vi "Initialize.vi"(8 "error in (no error)":errorcluster, 9 "Reset (True)":bool=TRUE, 10 "ID Query (True)":bool=TRUE, 11 "VISA resource name":refnum<visa-resource-name>) -> (0 "error out":errorcluster, 3 "VISA resource name out":refnum<visa-resource-name>)   [LabVIEW 2015, in "ZhiYuan ZDS Series for TCP.lvlib"]
doc: "Establishes communication with the instrument and optionally performs an instrument identification query and/or an instrument reset. It also places the instrument in a default state needed for other instrument driver operations. Therefore, call this VI before calling other instrument driver VIs for this instrument. Generally, you need to call the Initialize VI only once at the beginning of an application."
uses:
  ZhiYuan ZDS Series for TCP.lvlib
panel:
  # "(c) 2012 National Instruments.  ALL RIGHTS RESERVED."
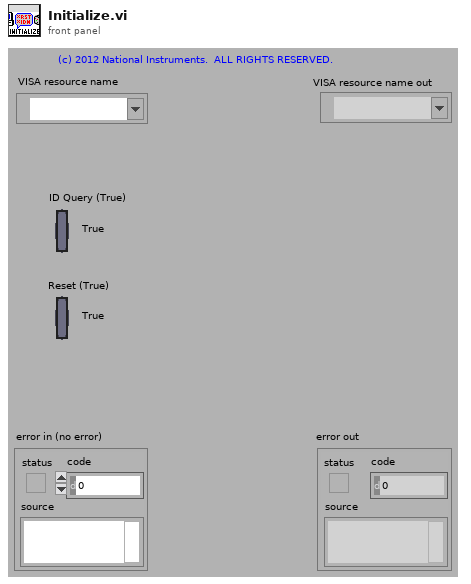
[diagram p1: front panel]
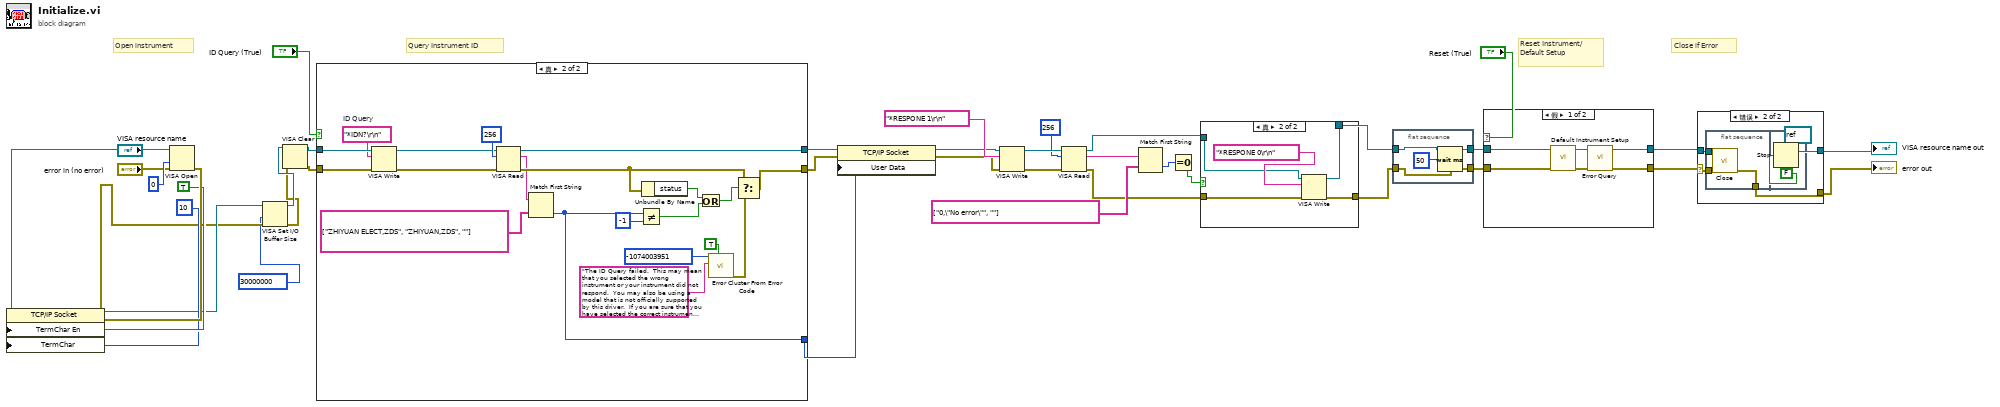
[diagram p0: block diagram]
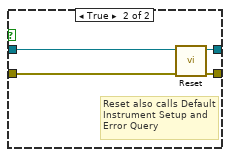
[diagram p4: hidden frame]
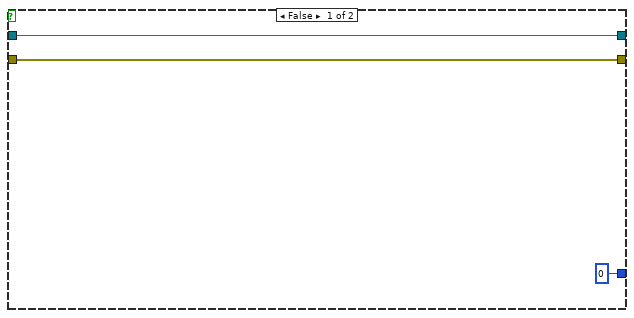
[diagram p5: hidden frame]
diagram:
  # "Close if Error"
  # "Query Instrument ID"
  # "Reset Instrument/\nDefault Setup"
  # "Open instrument"
  n1 = VISA Open(access mode=u32 0, error in (no error)="error in (no error)", VISA resource name="VISA resource name") -> (VISA resource name=w31:refnum<visa-resource-name>, error out=w30:errorcluster)  [unwired: 2 in]
  n2 = property class="TCP/IP Socket"(reference=w31, error in=w30, "TermChar En"=TRUE ("Message Based Settings:Termination Character Enable"), "TermChar"=u8 10 ("Message Based Settings:Termination Character")) -> (reference out=w23:refnum<visa-resource-name>, error out=w21:errorcluster)
  n3 = VISA Set I/O Buffer Size(VISA resource name=w23, size (4096)=30000000, error in (no error)=w21) -> (VISA resource name out=w22:refnum<visa-resource-name>, error out=w20:errorcluster)  [unwired: 1 in]
  n4 = VISA Clear(VISA resource name=w22, error in (no error)=w20) -> (VISA resource name out=w36:refnum<visa-resource-name>, error out=w35:errorcluster)
  n5 = case shown="真" "ID Query (True)" {
    tunnel: [w41 w62] -> w33
    tunnel: [w42 w59] -> w34
    tunnel: w36 -> [w42 w60]
    tunnel: w35 -> [w41 w61]
    tunnel: [0 ("index") w45] -> w32
    frame False {
    }
    frame True {
      w57 = "*IDN?\r\n"  # ID Query
      n6 = VISA Write(VISA resource name=w60, write buffer=w57, error in (no error)=w61) -> (VISA resource name out=w44:refnum<visa-resource-name>, error out=w43:errorcluster)  [unwired: 1 out]
      n7 = VISA Read(VISA resource name=w44, byte count=u32 256, error in (no error)=w43) -> (VISA resource name out=w59:refnum<visa-resource-name>, read buffer=w47:string, error out=w52:errorcluster)  [unwired: 1 out]
      n8 = Match First String(2:string[] ["ZHIYUAN ELECT,ZDS", "ZHIYUAN,ZDS", ""], 3:w47) -> (0:w45:i32)  [unwired: 1 out]
      n9 = Not Equal?(x=w45, y=-1) -> (x != y?=w50:bool)
      n10 = Unbundle By Name(w52) -> ("status"=w51:bool)
      n11 = Or(x=w51, y=w50) -> (x .or. y?=w49:bool)
      n12 = call <vilib>:"Error Cluster From Error Code.vi"("show call chain? (False)"=TRUE, "error message (\"\")"="The ID Query failed.  This may mean that you selected the wrong instrument or your instrument did not respond.  You may also be using a model that is not officially supported by this driver.  If you are sure that you have selected the correct instrument and it is responding, try disabling the ID Query." ("Source (VI Name)"), "error code (0)"=-1074003951 ("Code")) -> ("error out"=w56:errorcluster)  [unwired: 6 in]
      n13 = Select(t=w52, s=w49, f=w56) -> (s? t:f=w62:errorcluster)
    }
  }
  n14 = property on="Property Node" class="TCP/IP Socket"(reference=w34, error in=w33, "User Data"=w32) -> (reference out=w8:refnum<visa-resource-name>, error out=w7:errorcluster)
  n15 = VISA Write(VISA resource name=w8, write buffer="*RESPONE 1\r\n" ("Error Query Command"), error in (no error)=w7) -> (VISA resource name out=w17:refnum<visa-resource-name>, error out=w11:errorcluster)  [unwired: 1 out]
  n16 = VISA Read(VISA resource name=w17, byte count=u32 256 ("Bytes"), error in (no error)=w11) -> (VISA resource name out=w10:refnum<visa-resource-name>, read buffer=w14:string, error out=w9:errorcluster)  [unwired: 1 out]
  n17 = Match First String(2:string[] ["0,\"No error\"", ""], 3:w14) -> (0:w13:i32)  [unwired: 1 out]
  n18 = Equal To 0?(x=w13) -> (x = 0?=w12:bool)
  n19 = case shown="真" w12 {
    tunnel: w10 -> [w64 w68]
    tunnel: w9 -> [w63 w67]
    tunnel: [w63 w66] -> w6
    tunnel: [w64 w65] -> w5
    frame False {
    }
    frame True {
      n20 = VISA Write(VISA resource name=w68, write buffer="*RESPONE 0\r\n" ("Error Query Command"), error in (no error)=w67) -> (VISA resource name out=w65:refnum<visa-resource-name>, error out=w66:errorcluster)  [unwired: 1 out]
    }
  }
  n21 = flat-sequence {
    tunnel: w5 -> [w71]
    tunnel: w6 -> [w70]
    tunnel: [w71] -> w25
    tunnel: [w70] -> w24
    frame #0 {
      n22 = Wait (ms)(milliseconds to wait=u32 50 ("等待时间（毫秒）")) -> ()  [unwired: 1 out]
    }
  }
  n23 = case shown="假" "Reset (True)" {
    tunnel: w24 -> [w77 w79]
    tunnel: [w74 w82] -> w3
    tunnel: w25 -> [w78 w80]
    tunnel: [w75 w81] -> w4
    frame False {
      n24 = call "Default Instrument Setup.vi"("error in (no error)"=w77, "VISA resource name"=w78) -> ("error out"=w73:errorcluster, "VISA resource name out"=w76:refnum<visa-resource-name>)  [unwired: 8 in]
      n25 = call "Error Query.vi"("error in (no error)"=w73, "VISA resource name"=w76) -> ("error out"=w74:errorcluster, "VISA resource name out"=w75:refnum<visa-resource-name>)  [unwired: 6 in, 2 out]
    }
    frame True {
      # "Reset also calls Default Instrument Setup and Error Query"
      n26 = call "Reset.vi"("error in (no error)"=w79, "VISA resource name"=w80) -> ("error out"=w82:errorcluster, "VISA resource name out"=w81:refnum<visa-resource-name>)  [unwired: 8 in]
    }
  }
  n27 = case shown="错误" w3 {
    selector: w3 -> [w83 w87]
    tunnel: [w84 refnum<visa-resource-name> refnum ("VISA resource name out")] -> w2
    tunnel: w4 -> [w84 w86]
    tunnel: [w83 w85] -> w1
    frame No Error {
    }
    frame Error {
      n28 = flat-sequence {
        tunnel: w87 -> [w91]
        tunnel: w86 -> [w90]
        tunnel: [w89] -> w85
        frame #0 {
          n29 = call "Close.vi"("error in (no error)"=w91, "VISA resource name"=w90) -> ("error out"=w89:errorcluster)  [unwired: 9 in]
        }
        frame #1 {
          n30 = Stop(stop? (T)=FALSE) -> ()
        }
      }
    }
  }
  "VISA resource name out" <- w2
  "error out" <- w1
